vi "Write Page Enabled State.vi"(5 "Page Enabled State":T1(ring), 9 "Page in":refnum<class "Page.lvclass">) -> (3 "Page out":refnum<class "Page.lvclass">)   [LabVIEW 2014, in "Raspberry Pi Compatible Compiler for LabVIEW.lvlib" / "Page.lvclass"]
uses:
  Page.lvclass
  Page.lvclass/Page.ctl
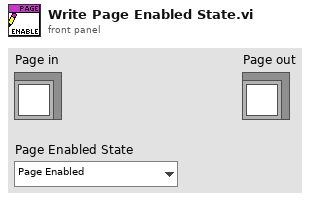
[diagram p1: front panel]
types:
  T1 = enum32{"Page Enabled", "Page Disabled", "Page Disabled & Grayed"}
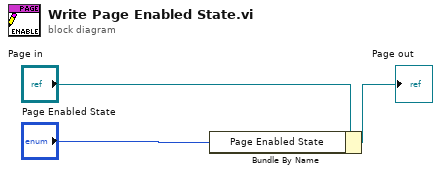
[diagram p0: block diagram]
diagram:
  n1 = Bundle By Name(cluster="Page in", "Page Enabled State"="Page Enabled State") -> (→"Page out":refnum<class "Page.lvclass">)
